vi "Get Slave Info.vi"(8 "error in (no error)":errorcluster, 11 "Master Device in":refnum<class "Master Device.lvclass">) -> (0 "error out":errorcluster, 2 "Slave Info":T1, 3 "Master Device out":refnum<class "Master Device.lvclass">)   [LabVIEW 2013, in "Master Device.lvclass"]
uses:
  Master Device.lvclass
  TypeDefs/SlaveInfo.ctl
  TypeDefs/RampInfo.ctl
  Master Device.lvclass/Master Device.ctl
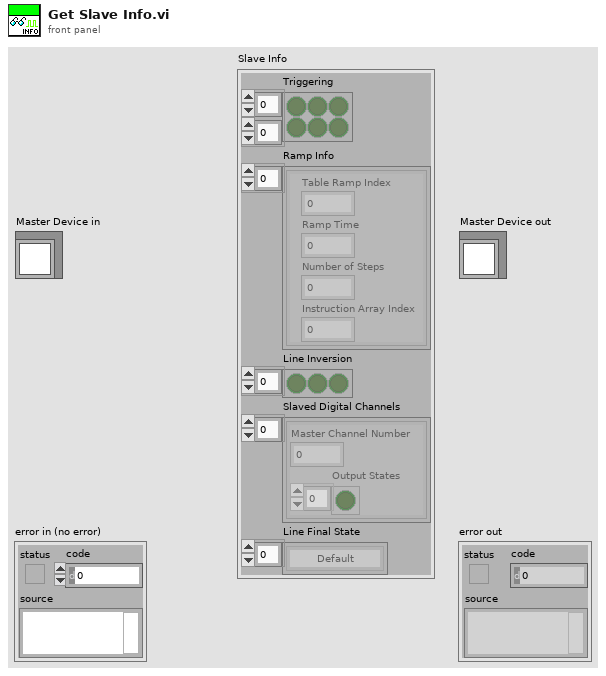
[diagram p1: front panel]
types:
  T1 = typedef "SlaveInfo.ctl" = cluster{"Triggering":bool[][], "Ramp Info":T2[], "Line Inversion":bool[], "Slaved Digital Channels":cluster{"Master Channel Number":i32, "Output States":bool[]}[], "Line Final State":enum16{"Default", "High", "Low", "Same"}[]}
  T2 = typedef "RampInfo.ctl" = cluster{"Table Ramp Index":i32, "Ramp Time":dbl, "Number of Steps":i32, "Instruction Array Index":i32}
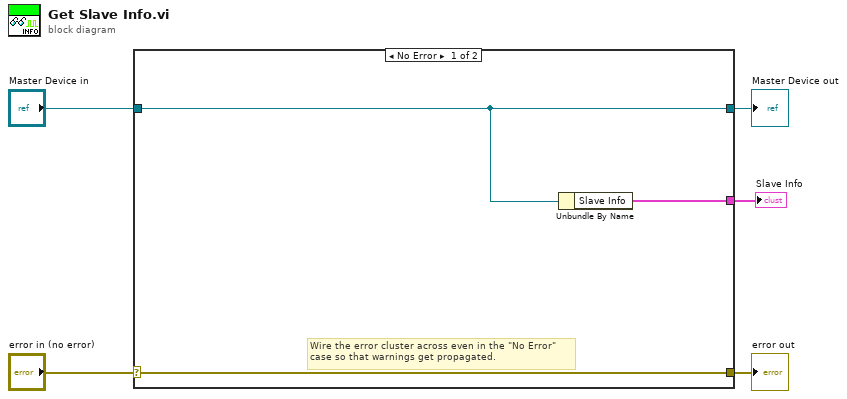
[diagram p0: block diagram]
diagram:
  n1 = case shown="No Error" "error in (no error)" {
    selector: "error in (no error)" -> [w8 w10]
    tunnel: [w8 w10] -> w4
    tunnel: [w7 w9] -> w2
    tunnel: "Master Device in" -> [w7 w9]
    tunnel: [w6 _] -> w1
    frame No Error {
      # "Wire the error cluster across even in the \"No Error\"\ncase so that warnings get propagated."
      n2 = Unbundle By Name(w7) -> ("Slave Info"=w6:T1)
    }
    frame Error {
    }
  }
  "error out" <- w4
  "Master Device out" <- w2
  "Slave Info" <- w1
